vi "預知保養設定讀取.vi"() -> ()   [LabVIEW 2019]
uses:
  LLB/Commonly VI/Main Glb.vi
  LLB/Commonly VI.lvlib
panel:
  out "測高使用次數":i32
  out "S4探針使用次數":i32
  out "S3探針使用次數":i32
  out "熱熔使用次數":i32
  out "焊接使用次數":i32
  out "S2探針使用次數":i32
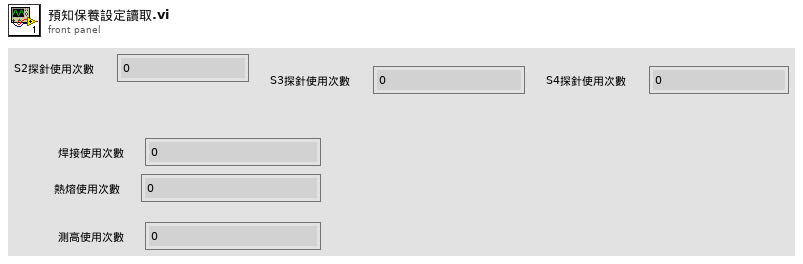
[diagram p1: front panel]
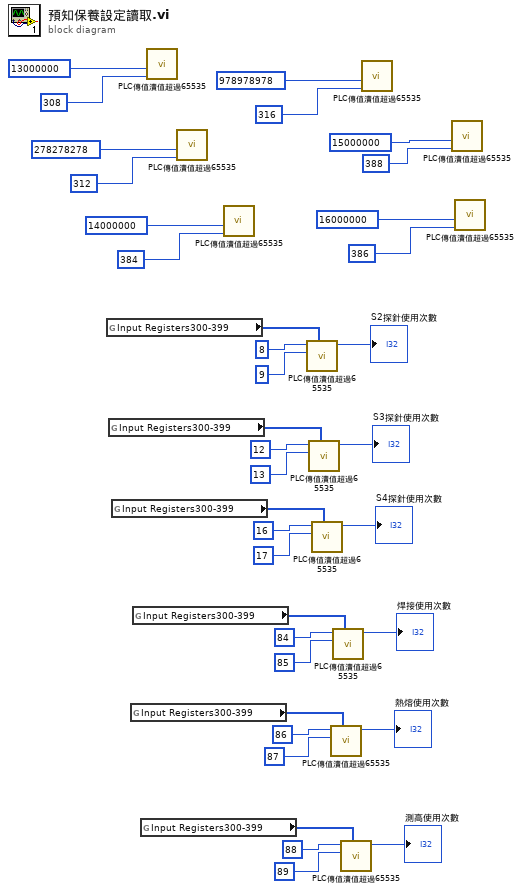
[diagram p0: block diagram]
diagram:
  n1 = global read "Main Glb.vi" "Input Registers300-399"() -> (w36:u16[])
  n2 = global read "Main Glb.vi" "Input Registers300-399"() -> (w9:u16[])
  n3 = global read "Main Glb.vi" "Input Registers300-399"() -> (w8:u16[])
  n4 = global read "Main Glb.vi" "Input Registers300-399"() -> (w28:u16[])
  n5 = global read "Main Glb.vi" "Input Registers300-399"() -> (w29:u16[])
  n6 = global read "Main Glb.vi" "Input Registers300-399"() -> (w1:u16[])
  n7 = call "PLC傳值瀆值超過65535.vi"("Out starting address"=u16 308, "Out輸入值"=u32 13000000) -> ()  [unwired: 9 in, 1 out]
  n8 = call "PLC傳值瀆值超過65535.vi"("Out starting address"=u16 312, "Out輸入值"=u32 278278278) -> ()  [unwired: 9 in, 1 out]
  n9 = call "PLC傳值瀆值超過65535.vi"("Out starting address"=u16 384, "Out輸入值"=u32 14000000) -> ()  [unwired: 9 in, 1 out]
  n10 = call "PLC傳值瀆值超過65535.vi"("Input Registers"=w36, "Read PLC Reg Index1"=9 ("Read PLC Reg Index0"), "Read PLC Reg Index0"=8) -> ("Receive PLC Data"=→"S2探針使用次數":i32)  [unwired: 8 in]
  n11 = call "PLC傳值瀆值超過65535.vi"("Input Registers"=w9, "Read PLC Reg Index1"=13 ("Read PLC Reg Index0"), "Read PLC Reg Index0"=12) -> ("Receive PLC Data"=→"S3探針使用次數":i32)  [unwired: 8 in]
  n12 = call "PLC傳值瀆值超過65535.vi"("Input Registers"=w8, "Read PLC Reg Index1"=17 ("Read PLC Reg Index0"), "Read PLC Reg Index0"=16) -> ("Receive PLC Data"=→"S4探針使用次數":i32)  [unwired: 8 in]
  n13 = call "PLC傳值瀆值超過65535.vi"("Input Registers"=w28, "Read PLC Reg Index1"=87 ("Read PLC Reg Index0"), "Read PLC Reg Index0"=86) -> ("Receive PLC Data"=→"熱熔使用次數":i32)  [unwired: 8 in]
  n14 = call "PLC傳值瀆值超過65535.vi"("Input Registers"=w29, "Read PLC Reg Index1"=85 ("Read PLC Reg Index0"), "Read PLC Reg Index0"=84) -> ("Receive PLC Data"=→"焊接使用次數":i32)  [unwired: 8 in]
  n15 = call "PLC傳值瀆值超過65535.vi"("Input Registers"=w1, "Read PLC Reg Index1"=89 ("Read PLC Reg Index0"), "Read PLC Reg Index0"=88) -> ("Receive PLC Data"=→"測高使用次數":i32)  [unwired: 8 in]
  n16 = call "PLC傳值瀆值超過65535.vi"("Out starting address"=u16 316, "Out輸入值"=u32 978978978) -> ()  [unwired: 9 in, 1 out]
  n17 = call "PLC傳值瀆值超過65535.vi"("Out starting address"=u16 388, "Out輸入值"=u32 15000000) -> ()  [unwired: 9 in, 1 out]
  n18 = call "PLC傳值瀆值超過65535.vi"("Out starting address"=u16 386, "Out輸入值"=u32 16000000) -> ()  [unwired: 9 in, 1 out]
